vi "ZeroMQTest.vi"() -> ()   [LabVIEW 2018]
doc: "Test VI for running the example code.\nExposes the 2 example classes, and keeps the communication alive for messages from the other language."
uses:
  Serializers/JSONJKI_class/JSONJKI.lvclass
  C:/VIT/VIT-Reuse/Examples/RemoteLabviewInterface/Serializers/Serializer_class/Serializer.lvclass
  Serializers/JSONJDP_class/JSONJDP.lvclass
  Published Classes/Console_class/Console.lvclass
  Published Classes/PerformanceTest_class/PerformanceTest.lvclass
  Executer_class/Executer.lvclass
  Communication/ZeroMQ_class/ZeroMQ.lvclass
panel:
  out "Running":i32
  in  "Start Button":bool
  in  "IP address":string
  in  "Port":string="5555"
  out "error out":errorcluster
  in  "Stop Button":bool
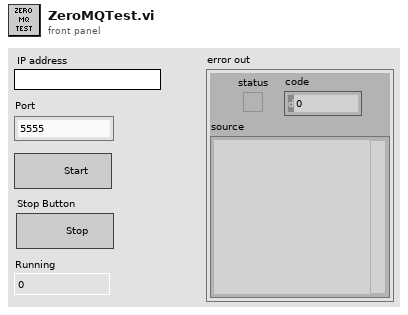
[diagram p1: front panel]
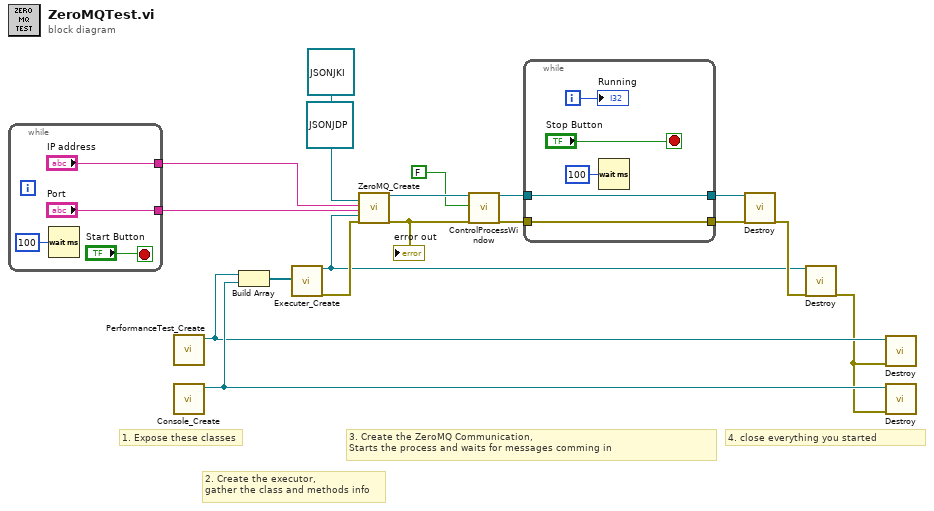
[diagram p0: block diagram]
diagram:
  (unwired) refnum<class "JSONJDP.lvclass"> refnum ("JSONJDP")
  # "4. close everything you started"
  # "3. Create the ZeroMQ Communication, \nStarts the process and waits for messages comming in"
  # "2. Create the executor, \ngather the class and methods info"
  # "1. Expose these classes"
  n1 = while {
    tunnel: ["IP address"] -> w8
    tunnel: ["Port"] -> w6
    stop <- "Start Button" stop-if-true
    n2 = Wait (ms)(milliseconds to wait=u32 100) -> ()  [unwired: 1 out]
  }
  n3 = call "PerformanceTest_Create.vi"() -> ("reference out"=w3:refnum<class "PerformanceTest.lvclass">)  [unwired: 10 in, 1 out]
  n4 = call "Console_Create.vi"() -> ("reference out"=w5:refnum<class "Console.lvclass">)  [unwired: 10 in, 1 out]
  n5 = Build Array(w3, w5) -> (w4:refnum<class>[])
  n6 = call "Executer_Create.vi"("Classes"=w4) -> ("reference out"=w7:refnum<class "Executer.lvclass">, "error out"=w15:errorcluster)  [unwired: 17 in]
  n7 = call "ZeroMQ_Create.vi"("Serializer"=refnum<class "JSONJKI.lvclass"> refnum ("JSONJKI"), "IP address"=w8, "Port"=w6, "Executor"=w7, "error in (no error)"=w15) -> ("reference out"=w17:refnum<class "ZeroMQ.lvclass">, "error out"=w16:errorcluster)  [unwired: 13 in]
  "error out" <- w16
  n8 = call "ControlProcessWindow.vi"("reference in"=w17, "ShowProcessWindow"=FALSE, "error in (no error)"=w16) -> ("reference out"=w13:refnum<class "ZeroMQ.lvclass">, "error out"=w9:errorcluster)  [unwired: 15 in]
  n9 = while {
    tunnel: [w24] -> w12
    tunnel: w13 -> [w24]
    tunnel: [w23] -> w11
    tunnel: w9 -> [w23]
    i -> [w22]
    stop <- "Stop Button" stop-if-true
    n10 = Wait (ms)(milliseconds to wait=u32 100) -> ()  [unwired: 1 out]
    "Running" <- w22
  }
  n11 = call-dynamic "Destroy.vi"("reference in"=w12, "error in (no error)"=w11) -> ("error out"=w10:errorcluster)  [unwired: 16 in, 1 out]
  n12 = call-dynamic "Destroy.vi"("reference in"=w7, "error in (no error)"=w10) -> ("error out"=w2:errorcluster)  [unwired: 16 in, 1 out]
  n13 = call-dynamic "Destroy.vi"("error in (no error)"=w2, "reference in"=w3) -> ()  [unwired: 8 in, 2 out]
  n14 = call-dynamic "Destroy.vi"("error in (no error)"=w2, "reference in"=w5) -> ()  [unwired: 8 in, 2 out]
